vi "Test LargeScrollbar.vi"() -> ()   [LabVIEW 2015, in "LargeScrollbar.lvclass"]
doc: "<b> </b> <b> </b>\n©2016 Q Software Innovations, LLC (QSI)\nwritten by Quentin Alldredge\nproduced in LabVIEW 2015\n\nsupport@qsoftwareinnovations.com\nwww.qsoftwareinnovations.com\n\nAll rights reserved.\n\nRedistribution and use in source and binary forms, with or without modification, are permitted provided that the following conditions are met:\n\n * Redistributions of source code must retain the above copyright notice, this list of conditions and the following disclaimer.\n * Redistributions in binary form must reproduce the above copyright notice, this list of conditions and the following disclaimer in the documentation and/or other materials provided with the distribution.\n * Neither the name of Q Software Innovations, LLC. nor the names of its contributors may be used to endorse or promote products derived from this software without specific prior written permission.\n\nTHIS SOFTWARE IS PROVIDED BY THE COPYRIGHT HOLDERS AND CONTRIBUTORS \"AS IS\" AND ANY EXPRESS OR IMPLIED WARRANTIES, INCLUDING, BUT NOT LIMITED TO, THE IMPLIED WARRANTIES OF MERCHANTABILITY AND FITNESS FOR A PARTICULAR PURPOSE ARE DISCLAIMED. IN NO EVENT SHALL THE COPYRIGHT OWNER OR CONTRIBUTORS BE LIABLE FOR ANY DIRECT, INDIRECT, INCIDENTAL, SPECIAL, EXEMPLARY, OR CONSEQUENTIAL DAMAGES (INCLUDING, BUT NOT LIMITED TO, PROCUREMENT OF SUBSTITUTE GOODS OR SERVICES; LOSS OF USE, DATA, OR PROFITS; OR BUSINESS INTERRUPTION) HOWEVER CAUSED AND ON ANY THEORY OF LIABILITY, WHETHER IN CONTRACT, STRICT LIABILITY, OR TORT (INCLUDING NEGLIGENCE OR OTHERWISE) ARISING IN ANY WAY OUT OF THE USE OF THIS SOFTWARE, EVEN IF ADVISED OF THE POSSIBILITY OF SUCH DAMAGE."
uses:
  LargeScrollbar.lvclass
  UpArrow.ctl
  DownArrow.ctl
  LeftArrow.ctl
  RightArrow.ctl
panel:
  in  "Horizontal Scrollbar Max":u32
  in  "Vertical Scrollbar Max":u32
  out "Horizontal Scrollbar Value":u32
  in  "Horizontal Scrollbar":T3 {"Slide" scale=0.0..1000.0}
  out "Vertical Scrollbar Value":u32
  in  "Vertical Scrollbar":T6
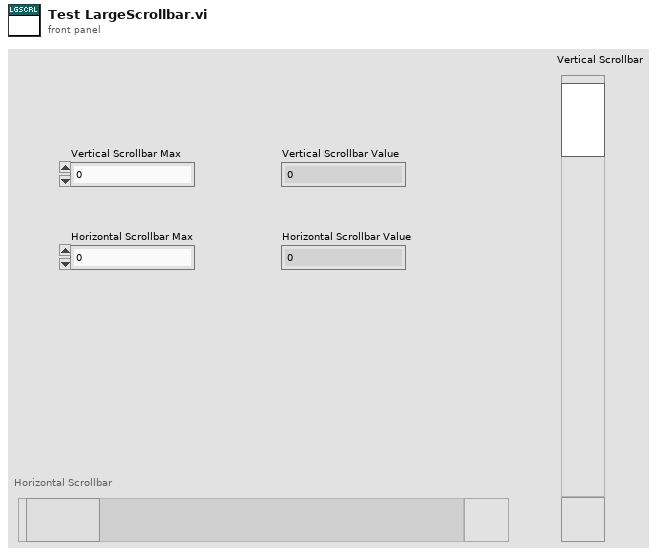
[diagram p1: front panel]
types:
  T1 = typedef "LargeScrollbar.lvclass/LeftArrow.ctl" = bool
  T2 = typedef "LargeScrollbar.lvclass/RightArrow.ctl" = bool
  T3 = cluster{"LeftButton":T1, "Slide":u32, "RightButton":T2}
  T4 = typedef "LargeScrollbar.lvclass/UpArrow.ctl" = bool
  T5 = typedef "LargeScrollbar.lvclass/DownArrow.ctl" = bool
  T6 = cluster{"UpButton":T4, "Slide":u32, "DownButton":T5}
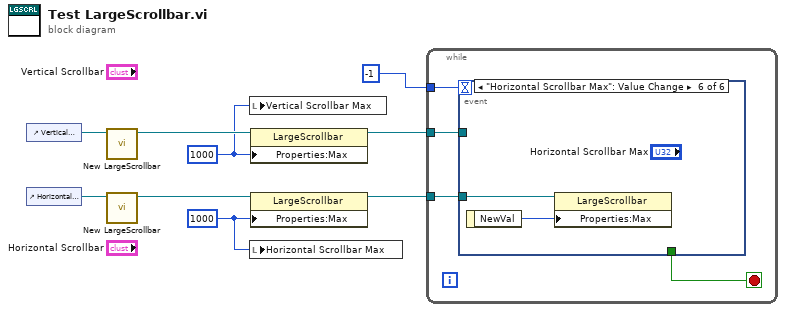
[diagram p0: block diagram]
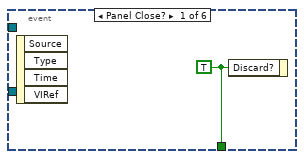
[diagram p2: hidden frame]
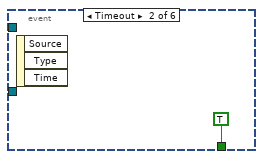
[diagram p3: hidden frame]
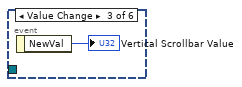
[diagram p4: hidden frame]
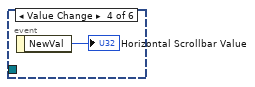
[diagram p5: hidden frame]
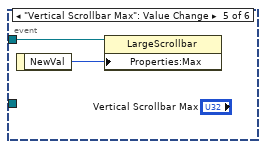
[diagram p6: hidden frame]
diagram:
  w4 = u32 1000 ("Max")
  w3 = u32 1000 ("Max")
  n1 = control-ref of="Vertical Scrollbar"() -> (w9:refnum<vi>)
  n2 = control-ref of="Horizontal Scrollbar"() -> (w5:refnum<vi>)
  n3 = call "New LargeScrollbar.vi"("Reference"=w9) -> ("LargeScrollbar out"=w8:refnum<class "LargeScrollbar.lvclass">)  [unwired: 9 in, 1 out]
  n4 = call "New LargeScrollbar.vi"("Reference"=w5) -> ("LargeScrollbar out"=w6:refnum<class "LargeScrollbar.lvclass">)  [unwired: 9 in, 1 out]
  n5 = local write "Vertical Scrollbar Max"(w3) -> ()
  n6 = local write "Horizontal Scrollbar Max"(w4) -> ()
  n7 = property class="LargeScrollbar"(reference=w8, "Properties:Max"=w3) -> (reference out=w7:refnum<class "LargeScrollbar.lvclass">)  [unwired: 1 in, 1 out]
  n8 = property class="LargeScrollbar"(reference=w6, "Properties:Max"=w4) -> (reference out=w1:refnum<class "LargeScrollbar.lvclass">)  [unwired: 1 in, 1 out]
  n9 = while {
    tunnel: w7 -> [w13]
    tunnel: w1 -> [w11]
    tunnel: -1 -> [w10]
    stop <- w12 stop-if-true
    n10 = event shown="[5] \"Horizontal Scrollbar Max\": Value Change" {
      selector: _ -> [_ _ _ _ _ _]
      dyn-events: _ -> [_ _ _ _ _ _]
      timeout: w10 -> [_ _ _ _ _ _]
      tunnel: w13 -> [_ _ _ _ w18 _]
      tunnel: [w14 TRUE ("Discard?") _ _ _ _] -> w12
      tunnel: w11 -> [_ _ _ _ _ w21]
      event Panel Close? {
        w14 = TRUE ("Discard?")
        n11 = event-data() -> ()  [unwired: 1 in, 4 out]
        n12 = event-data("Discard?"=w14) -> ()  [unwired: 1 in, 1 out]
      }
      event Timeout {
        n13 = event-data() -> ()  [unwired: 1 in, 3 out]
      }
      event "Vertical Scrollbar.Slide": Value Change {
        n14 = event-data() -> ("NewVal"=→"Vertical Scrollbar Value":u32)  [unwired: 1 in]
      }
      event "Horizontal Scrollbar.Slide": Value Change {
        n15 = event-data() -> ("NewVal"=→"Horizontal Scrollbar Value":u32)  [unwired: 1 in]
      }
      event "Vertical Scrollbar Max": Value Change {
        n16 = event-data() -> ("NewVal"=w19:u32)  [unwired: 1 in]
        n17 = property class="LargeScrollbar"(reference=w18, "Properties:Max"=w19) -> ()  [unwired: 1 in, 2 out]
      }
      event "Horizontal Scrollbar Max": Value Change {
        n18 = event-data() -> ("NewVal"=w20:u32)  [unwired: 1 in]
        n19 = property class="LargeScrollbar"(reference=w21, "Properties:Max"=w20) -> ()  [unwired: 1 in, 2 out]
      }
    }
  }
